vi "updateTestParameters.vi"(8 "error in (no error)":errorcluster, 10 "Test Parameters":T1 {"Max records per file" min=100 max=1000000; "Cycle profile"."Pause After" min=1.0 max=600.0 format="%.1f"; "Cycle profile"."Force Setpoint" min=-556.0 max=556.0 format="%.1f"; "Number of cycles for complete test" min=1}, 11 "Model in":refnum<class "Model.lvclass">) -> (0 "error out":errorcluster, 3 "Model out":refnum<class "Model.lvclass">)   [LabVIEW 2013, in "Model.lvclass"]
uses:
  Model.lvclass
  Configuration/Test Parameters.ctl
  Configuration/CycleProfileConfig.ctl
  Model.lvclass/Model.ctl
  ApplicationElements/TestMonitor/TestMonitor.lvclass/TestMonitor.ctl
  ApplicationElements/TestMonitor/TestMonitor.lvclass
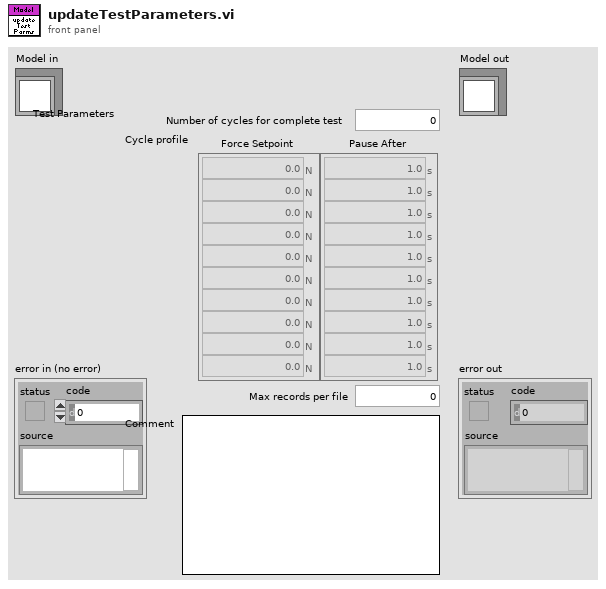
[diagram p1: front panel]
types:
  T1 = typedef "Test Parameters.ctl" = cluster{"Number of cycles for complete test":u32, "Cycle profile":T2, "Max records per file":u32, "Comment":string}
  T2 = typedef "CycleProfileConfig.ctl" = cluster{"Force Setpoint":dbl[unit][], "Pause After":dbl[unit][]}
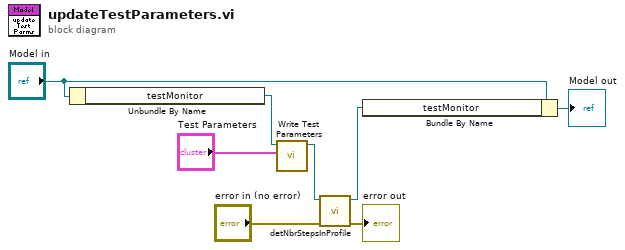
[diagram p0: block diagram]
diagram:
  n1 = Unbundle By Name("Model in") -> ("testMonitor"=w7:refnum<class "TestMonitor.lvclass">)
  n2 = call "Write Test Parameters.vi"("Test Parameters"="Test Parameters", "TestMonitor in"=w7) -> ("TestMonitor out"=w6:refnum<class "TestMonitor.lvclass">)  [unwired: 9 in]
  n3 = call "detNbrStepsInProfile.vi"("error in (no error)"="error in (no error)", "TestMonitor in"=w6) -> ("error out"=→"error out":errorcluster, "TestMonitor out"=w5:refnum<class "TestMonitor.lvclass">)  [unwired: 8 in]
  n4 = Bundle By Name(cluster="Model in", "testMonitor"=w5) -> (→"Model out":refnum<class "Model.lvclass">)
